vi "ATMonochromator_cancelCallback_logEvent_settingsAppliedLoop.vi"(8 "error in (no error)":errorcluster) -> (0 "error out":errorcluster, 3 "function return":i32)   [LabVIEW 2016, in "SALLV_ATMonochromator.lvlib"]
doc: "int ATMonochromator_shm_cancelCallback_logevent_settingsAppliedLoopLV();"
uses:
  SALLV_ATMonochromator.lvlib
  SALLV_ATMonochromator.so
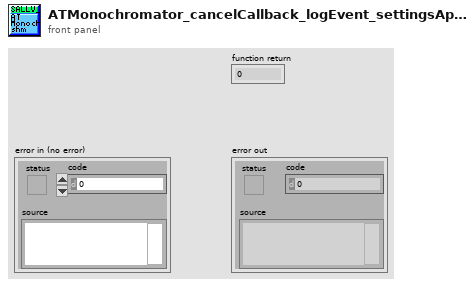
[diagram p1: front panel]
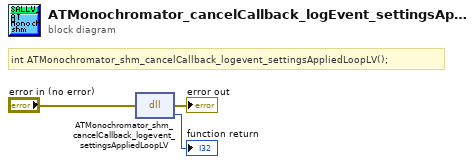
[diagram p0: block diagram]
diagram:
  # "int ATMonochromator_shm_cancelCallback_logevent_settingsAppliedLoopLV();"
  n1 = dll-call lib="home/harini/tcs/SALLV_ATMonochromator/SALLV_ATMonochromator.*" fn="ATMonochromator_shm_cancelCallback_logevent_settingsAppliedLoopLV"(error in="error in (no error)") -> (error out=→"error out":errorcluster, →"function return":i32)  [unwired: 2 in, 1 out]
